vi "PreviewMultiplePackageInstall.vi"(8 "Error In":errorcluster, 10 "Include Recommended?":bool, 11 "Packages":cluster{"Package":string, "Version":string}[](array[cluster])) -> (0 "Error Out":errorcluster, 2 "Install Command":string, 3 "Preview":string)   [LabVIEW 2019, in "CEPM.lvlib"]
uses:
  CEPM.lvlib
  <vilib>/Utility/sysdir.llb/System Directory Type.ctl
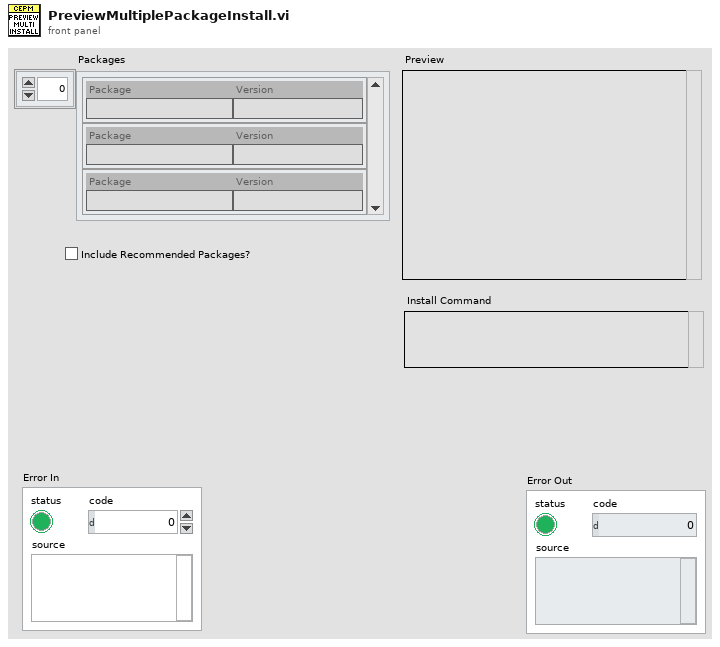
[diagram p1: front panel]
types:
  T1 = typedef "System Directory Type.ctl" = i32
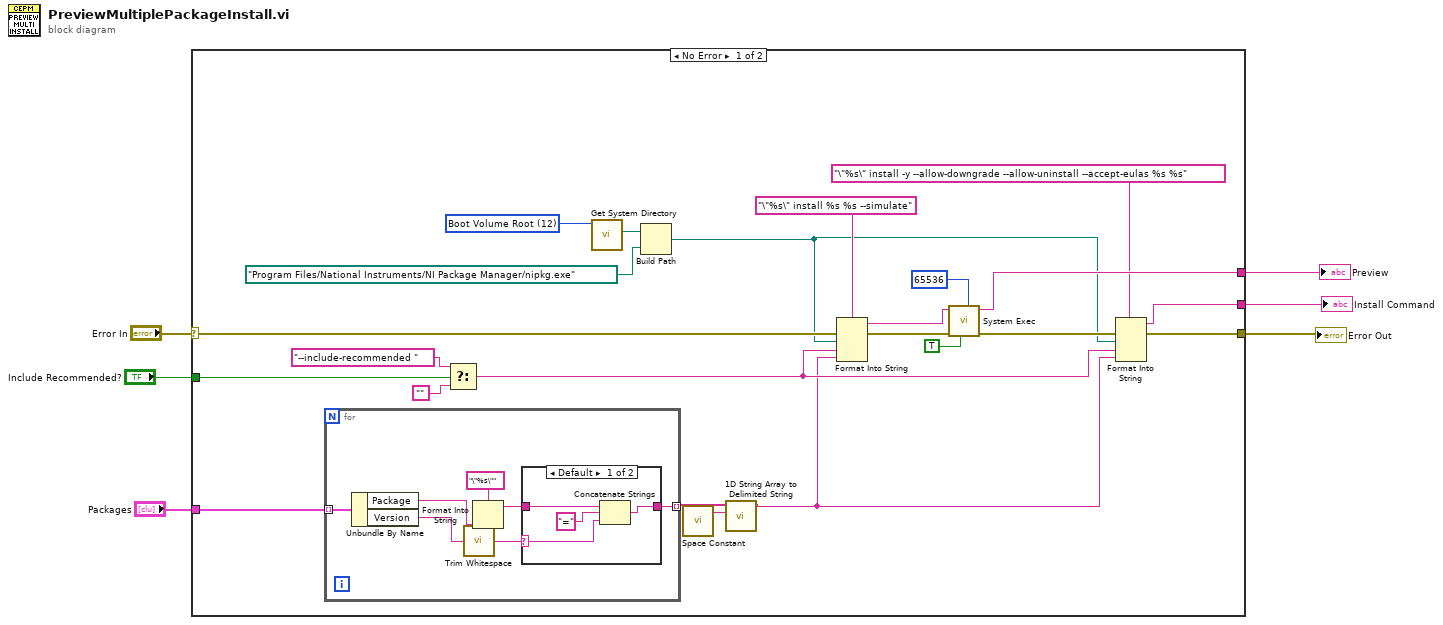
[diagram p0: block diagram]
diagram:
  n1 = case shown="No Error" "Error In" {
    selector: "Error In" -> [w29 w42]
    tunnel: [w15 w42] -> w5
    tunnel: [w20 _] -> w4
    tunnel: "Include Recommended?" -> [w17 _]
    tunnel: [w11 _] -> w2
    tunnel: "Packages" -> [w10 _]
    frame No Error {
      w25 = T1 12 items=["User Home"=0, "User Desktop"=1, "User Documents"=2, "User Application Data"=3, "User Preferences"=4, "User Temporary"=5, "Public Documents"=6, "Public Application Data"=7, "Public Preferences"=8, "Public Cache"=13, "System Core Libraries"=9, "System Installed Libraries"=10, "Application Files"=11, "Boot Volume Root"=12] ("system directory type")
      n2 = for {
        tunnel: [w35] -> w9 mode=indexing
        tunnel: w10 -> [w32] mode=indexing
        n3 = Unbundle By Name(w32) -> ("Package"=w31:string, "Version"=w30:string)
        n4 = call <vilib>:"Trim Whitespace.vi"("string"=w30) -> ("trimmed string"=w36:string)  [unwired: 1 in]
        n5 = Format Into String(format string="\"%s\"", w31) -> (resulting string=w33:string)  [unwired: 2 in, 1 out]
        n6 = case shown="Default" w36 {
          selector: w36 -> [w39 _]
          tunnel: w33 -> [w40 w41]
          tunnel: [w37 w41] -> w35
          frame Default {
            n7 = Concatenate Strings(w40, "=" ("string"), w39) -> (w37:string)
          }
          frame "" {
          }
        }
      }
      n8 = Select(t="--include-recommended ", s=w17, f="") -> (s? t:f=w13:string)
      n9 = call <vilib>:"Get System Directory.vi"("system directory type"=w25) -> ("system directory"=w26:path)  [unwired: 10 in]
      n10 = Build Path(base path=w26, name or relative path=path "Program Files/National Instruments/NI Package Manager/nipkg.exe" ("working directory")) -> (appended path=w14:path)
      n11 = call <vilib>:"Space Constant.vi"() -> ("String"=w8:string)
      n12 = call <vilib>:"1D String Array to Delimited String.vi"("delimiter"=w8, "string array"=w9) -> ("delimited string"=w7:string)  [unwired: 9 in]
      n13 = Format Into String(format string="\"%s\" install %s %s --simulate", error in=w29, w14, w13, w7) -> (resulting string=w23:string, error out=w28:errorcluster)  [unwired: 1 in]
      n14 = call <vilib>:"System Exec.vi"("expected output size  (4096)"=u32 65536, "run minimized? (F)"=TRUE, "error in (no error)"=w28, "command line"=w23) -> ("error out"=w16:errorcluster, "standard output"=w20:string)  [unwired: 4 in, 2 out]
      n15 = Format Into String(format string="\"%s\" install -y --allow-downgrade --allow-uninstall --accept-eulas %s %s", error in=w16, w14, w13, w7) -> (resulting string=w11:string, error out=w15:errorcluster)  [unwired: 1 in]
    }
    frame Error {
    }
  }
  "Error Out" <- w5
  "Preview" <- w4
  "Install Command" <- w2
